vi "Get baud rate.vi"(11 "BD Protocol 4.0 in":refnum<class "BD Protocol 4.0.lvclass">) -> (2 "baud rate":refnum<vi>, 3 "BD Protocol 4.0 out":refnum<class "BD Protocol 4.0.lvclass">)   [LabVIEW 2016, in "BD Protocol 4.0.lvlib" / "BD Protocol 4.0.lvclass"]
uses:
  BD Protocol 4.0.lvclass
  BD Protocol 4.0.lvclass/BD Protocol 4.0.ctl
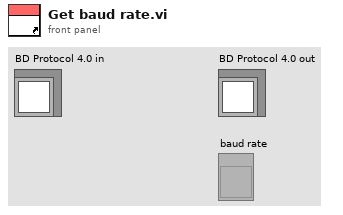
[diagram p1: front panel]
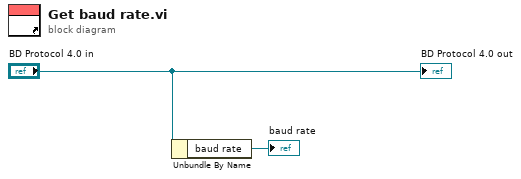
[diagram p0: block diagram]
diagram:
  n1 = Unbundle By Name("BD Protocol 4.0 in") -> ("baud rate"=→"baud rate":refnum<vi>)
  "BD Protocol 4.0 out" <- "BD Protocol 4.0 in"
